vi "GetVariablesTable.vi"(8 "error in (no error)":errorcluster, 9 "SignificantDigits (8)":u32=8, 10 "Format (SI notation)":T1(ring)=enum."SI notation", 11 "VariableManagerRef in":refnum<vi>) -> (0 "error out":errorcluster, 2 "VariableTable":string[][](array[string]), 3 "VariableManagerRef out":refnum<vi>)   [LabVIEW 2013, in "VariableManagerAPI.lvlib"]
doc: "Return a 2D array of string representing all variable definitions in the variable manager.\n\nBLANK|VariableName | DefaultValue | SequenceFunction | Sequence | InformIgorss"
uses:
  VariableManagerAPI.lvlib
  VariableManager/VariableManager.lvclass
  Variable/Variable.lvclass
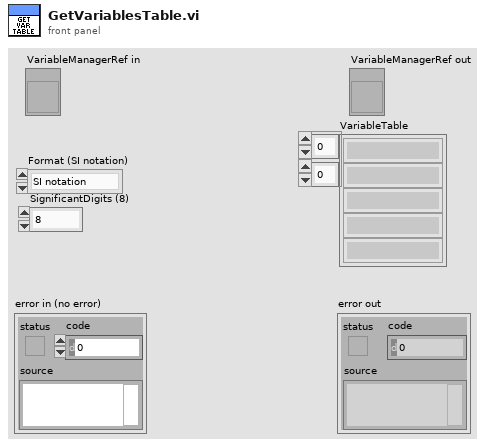
[diagram p1: front panel]
types:
  T1 = enum16{"Floating point", "Scientific SI", "Automatic SI", "SI notation"}
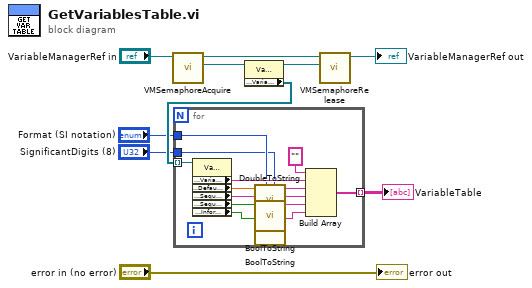
[diagram p0: block diagram]
diagram:
  n1 = call "VMSemaphoreAcquire.vi"("VariableManagerRef in"="VariableManagerRef in") -> ("VariableManager"=w7:refnum<class "VariableManager.lvclass">, "VariableManagerRef out"=w9:refnum<vi>)  [unwired: 7 in, 2 out]
  n2 = property class="VariableManager.lvclass"(reference=w7) -> (reference out=w6:refnum<class "VariableManager.lvclass">, "Accessors:Variables"=w5:refnum<class "Variable.lvclass">[])  [unwired: 1 in, 1 out]
  n3 = for {
    tunnel: w5 -> [w23] mode=indexing
    tunnel: [w17] -> w4 mode=indexing
    tunnel: "Format (SI notation)" -> [w12]
    tunnel: "SignificantDigits (8)" -> [w11]
    n4 = property class="Variable.lvclass"(reference=w23) -> ("Accessors:VariableName"=w21:string, "Accessors:DefaultValue"=w14:dbl, "Accessors:SequenceFunction"=w20:string, "Accessors:Sequence"=w16:bool, "Accessors:InformIgor"=w22:bool)  [unwired: 1 in, 2 out]
    n5 = call "DoubleToString.vi"("SignificantDigits (8)"=w11, "Format (SI notation)"=w12, "Double"=w14) -> ("String"=w13:string)  [unwired: 8 in]
    n6 = call "BoolToString.vi"("BooleanIn"=w16) -> ("String"=w19:string)  [unwired: 10 in]
    n7 = call "BoolToString.vi"("BooleanIn"=w22) -> ("String"=w18:string)  [unwired: 10 in]
    n8 = Build Array("" ("element"), w21, w13, w20, w19, w18) -> (w17:string[])
  }
  "VariableTable" <- w4
  n9 = call "VMSemaphoreRelease.vi"("VariableManager"=w6, "VariableManagerRef in"=w9) -> ("VariableManagerRef out"=→"VariableManagerRef out":refnum<vi>)  [unwired: 8 in, 1 out]
  "error out" <- "error in (no error)"
